vi "Nested Exist Wrapper.vi"(11 "Dev Actor in":refnum<class "Dev Actor.lvclass">) -> (2 "Nested Exist?":bool)   [LabVIEW 2021, in "Dev Actor.lvlib" / "Dev Actor.lvclass"]
uses:
  Dev Actor.lvclass
  Dev Actor.lvclass/Dev Actor.ctl
  LVCAM/LVCAM/Actor/Actor.lvclass
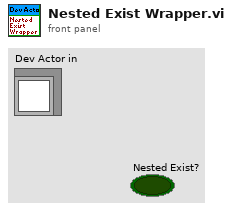
[diagram p1: front panel]
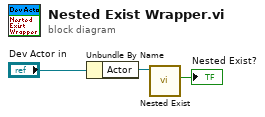
[diagram p0: block diagram]
diagram:
  n1 = Unbundle By Name("Dev Actor in") -> ("Actor"=w2:refnum<class "Actor.lvclass">)
  n2 = call-dynamic "Nested Exist.vi"("Actor in"=w2) -> ("Nested Exist?"=→"Nested Exist?":bool)  [unwired: 10 in]
